vi "IMAQdx Low-Level Grab Async with AVI Recording LV2012 NIVerified.vi"() -> ()   [LabVIEW 2012]
doc: "Demonstrates how to save acquired images to a AVI.\n\nIn this example a IMAQdx Acquisition (e.g. USB Webcams) is used to generate images that can be saved to a AVI file. But in general a AVI file can be generated off every series of IMAQ Images. Other IMAQ Image sources could be other IMAQ drivers (IMAQ, IMAQ I/O) or loading a series of images from disk."
uses:
  <vilib>/userdefined/High Color/IMAQdx.ctl
  <vilib>/vision/driver/IMAQdx.llb/IMAQdx Acquisition Mode.ctl
  <vilib>/vision/driver/IMAQdx.llb/IMAQdx Buffer Number Mode.ctl
  <vilib>/vision/driver/NI_Vision_Acquisition_Software.lvlib
  <resource>/objmgr/imaqdx.rc
panel:
  in  "stop":bool
  in  "Record":bool
  in  "Camera Name":T1
  out "Image":T2(plugin-control)
  out "Buffer Number":u32
  out "Event Overrun":bool
  in  "AVI File Path":path
  # "Overview: Demonstrates how to save acquired images to a AVI video\nRequirements: LabVIEW 2012 Base Development System  (or compatible)\n                             Vision Development Module 2012 (or compatible)\n                             NI-IMAQdx 4.0 (or compatible)\nInstructions: \n1. Select the path to the AVI file\n2. Select the camera name\n3. Run the VI\n4. Activate the Record button to start writing image frames to the AVI\n5. Release the button to stop recording"
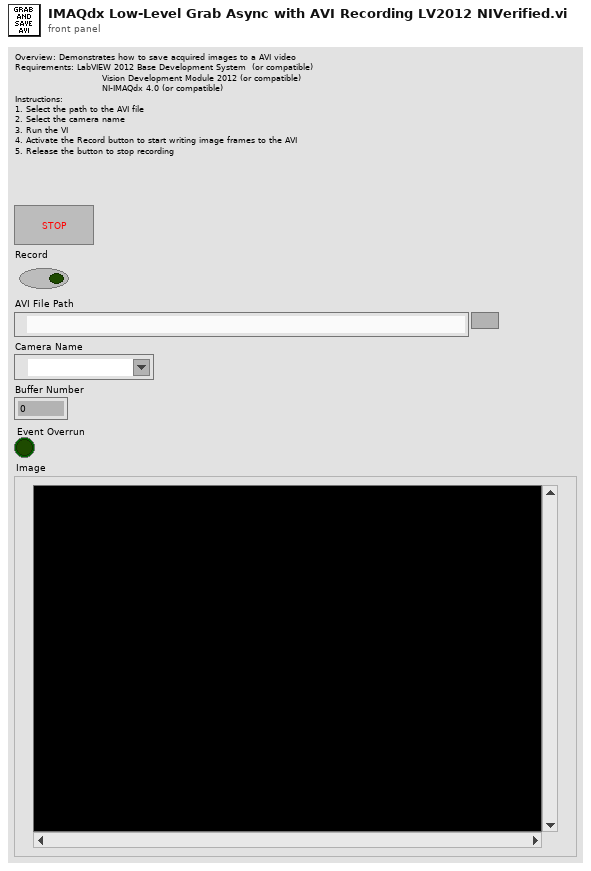
[diagram p1: front panel]
types:
  T1 = typedef "IMAQdx.ctl" = refnum<k21>
  T2 = typedef "IMAQ Image.ctl" = refnum<image>
  T3 = typedef "NI_Vision_Acquisition_Software.lvlib/IMAQdx Acquisition Mode.ctl" = enum32{"One Shot", "Continuous"}
  T4 = typedef "IMAQ AVI2 Refnum.ctl" = refnum<k20>
  T5 = typedef "NI_Vision_Acquisition_Software.lvlib/IMAQdx Buffer Number Mode.ctl" = enum32{"Next", "Last", "Buffer Number"}
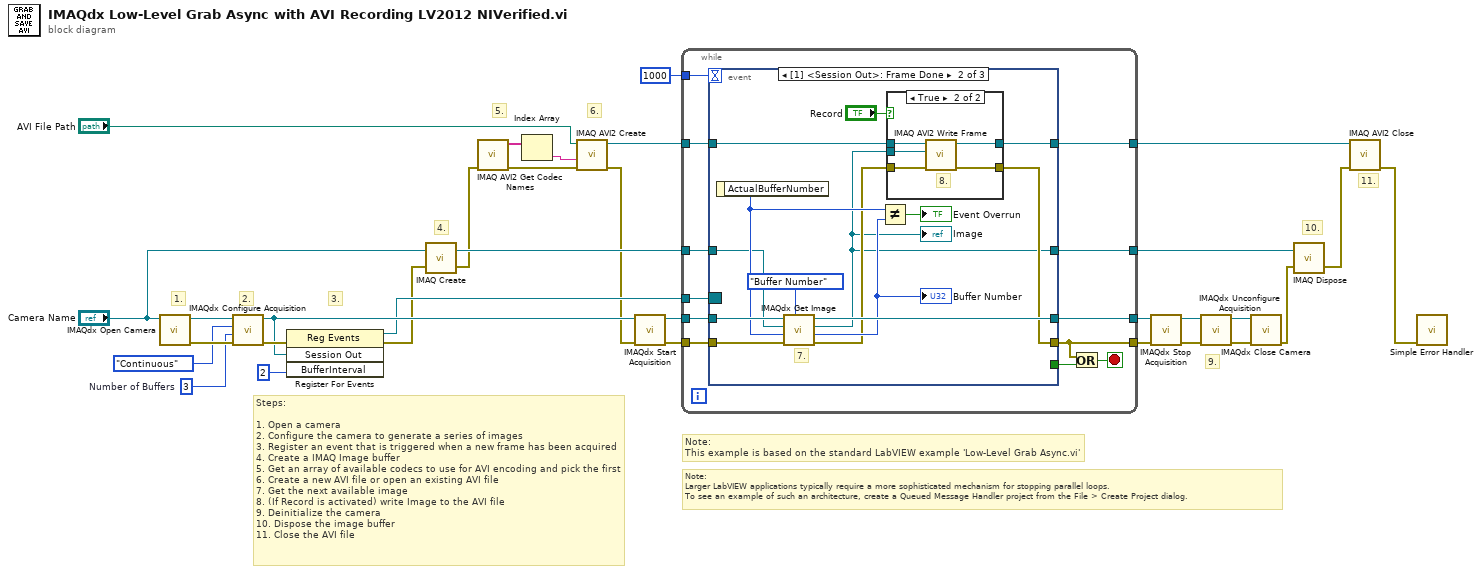
[diagram p0: block diagram]
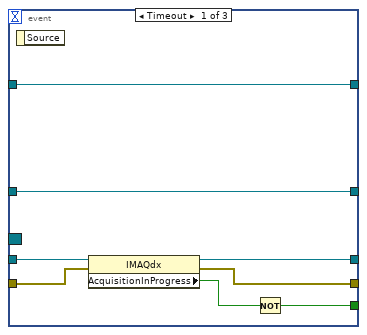
[diagram p2: hidden frame]
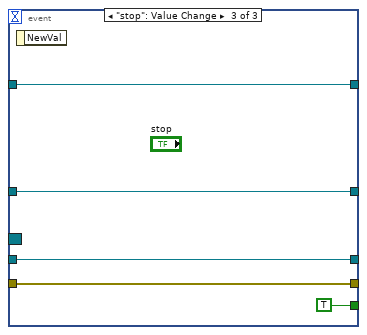
[diagram p4: hidden frame]
diagram:
  w26 = u32 3  # Number of Buffers
  # "Note:\nLarger LabVIEW applications typically require a more sophisticated mechanism for stopping parallel loops.\nTo see an example of such an architecture, create a Queued Message Handler project from the File > Create Project dialog."
  # "10."
  # "11."
  # "9."
  # "6."
  # "5."
  # "4."
  # "3."
  # "2."
  # "1."
  # "Note:\nThis example is based on the standard LabVIEW example 'Low-Level Grab Async.vi'"
  # "Steps:\n\n1. Open a camera\n2. Configure the camera to generate a series of images \n3. Register an event that is triggered when a new frame has been acquired\n4. Create a IMAQ Image buffer\n5. Get an array of available codecs to use for AVI encoding and pick the first\n6. Create a new AVI file or open an existing AVI file\n7. Get the next available image\n8. (If Record is activated) write Image to the AVI file\n9. Deinitialize the camera\n10. Dispose the image buffer\n11. Close the AVI file"
  n1 = call <vilib>:"IMAQdx Open Camera.vi"("Session In"="Camera Name") -> ("error out"=w28:errorcluster, "Session Out"=w30:T1)  [unwired: 2 in, 7 out]
  n2 = call <vilib>:"IMAQdx Configure Acquisition.vi"("error in"=w28, "Number of Buffers"=w26, "Continuous?"=IMAQdx_Acquisition_Mode."Continuous", "Session In"=w30) -> ("error out"=w19:errorcluster, "Session Out"=w18:T1)  [unwired: 6 out]
  n3 = register-events(error in=w19, w18, u32 2 ("BufferInterval")) -> (reference out=w16:refnum<event-registration>, error out=w14:errorcluster)  [unwired: 1 in]
  n4 = call "IMAQ Create"("Image Name"="Camera Name", "error in (no error)"=w14) -> ("New Image"=w32:T2, "error out"=w13:errorcluster)  [unwired: 2 in, 1 out]
  n5 = call "IMAQ AVI2 Get Codec Names"("error in (no error)"=w13) -> ("error out"=w9:errorcluster, "Codec Names"=w12:string[])  [unwired: 9 in]
  n6 = Index Array(array=w12) -> (element=w10:string)  [unwired: 1 in]
  n7 = call "IMAQ AVI2 Create"("error in (no error)"=w9, "Codec"=w10, "AVI Path"="AVI File Path") -> ("error out"=w7:errorcluster, "AVI Refnum"=w6:T4)  [unwired: 7 in]
  n8 = call <vilib>:"IMAQdx Start Acquisition.vi"("error in"=w7, "Session In"=w18) -> ("error out"=w8:errorcluster, "Session Out"=w29:T1)  [unwired: 8 out]
  n9 = while {
    tunnel: [w40] -> w24
    tunnel: w8 -> [w42]
    tunnel: w29 -> [w43]
    tunnel: [w37] -> w25
    tunnel: w32 -> [w41]
    tunnel: w16 -> [w39]
    tunnel: 1000 -> [w38]
    tunnel: w6 -> [w35]
    tunnel: [w34] -> w5
    tunnel: [w33] -> w3
    stop <- w44 stop-if-true
    n10 = event shown="[1] <Session Out>: Frame Done" {
      selector: w39 -> [_ _ _]
      dyn-events: _ -> [_ _ _]
      timeout: w38 -> [_ _ _]
      tunnel: w43 -> [w52 w66 w77]
      tunnel: w42 -> [w48 w65 w78]
      tunnel: w41 -> [w50 w54 w74]
      tunnel: [w49 w64 w77] -> w40
      tunnel: [w47 w56 w78] -> w37
      tunnel: [w45 _ TRUE] -> w36
      tunnel: w35 -> [w51 w59 w75]
      tunnel: [w51 w58 w75] -> w34
      tunnel: [w50 w53 w74] -> w33
      event Timeout {
        n11 = event-data() -> ()  [unwired: 2 out]
        n12 = property class="IMAQdx"(reference=w52, error in=w48) -> (reference out=w49:T1, error out=w47:errorcluster, "AcquisitionInProgress"=w46:bool)
        n13 = Not(x=w46) -> (.not. x?=w45:bool)
      }
      event event #0x0 {
        # "7."
        n14 = event-data() -> ("ActualBufferNumber"=w62:u32)  [unwired: 1 out]
        n15 = call <vilib>:"IMAQdx Get Image.vi"("Buffer Number Mode (Next)"=IMAQdx_Buffer_Number_Mode."Buffer Number" ("Buffer Number Mode"), "error in"=w65, "Buffer Number In"=w62, "Image In"=w54, "Session In"=w66) -> ("error out"=w57:errorcluster, "Buffer Number Out"=w61:u32, "Image Out"=w53:T2, "Session Out"=w64:T1)  [unwired: 3 out]
        "Image" <- w53
        "Buffer Number" <- w61
        n16 = Not Equal?(x=w62, y=w61) -> (x != y?=→"Event Overrun":bool)
        n17 = case shown="True" "Record" {
          tunnel: w59 -> [w67 w73]
          tunnel: [w67 w72] -> w58
          tunnel: w53 -> [_ w71]
          tunnel: w57 -> [w68 w70]
          tunnel: [w68 w69] -> w56
          frame False {
          }
          frame True {
            # "8."
            n18 = call "IMAQ AVI2 Write Frame"("error in (no error)"=w70, "Image"=w71, "AVI Refnum"=w73) -> ("error out"=w69:errorcluster, "AVI Refnum (duplicate)"=w72:T4)  [unwired: 6 in, 1 out]
          }
        }
      }
      event "stop": Value Change {
        n19 = event-data() -> ()  [unwired: 2 out]
      }
    }
    n20 = Or(x=w37, y=w36) -> (x .or. y?=w44:bool)
  }
  n21 = call <vilib>:"IMAQdx Stop Acquisition.vi"("error in"=w25, "Session In"=w24) -> ("error out"=w20:errorcluster, "Session Out"=w21:T1)  [unwired: 8 out]
  n22 = call <vilib>:"IMAQdx Unconfigure Acquisition.vi"("error in"=w20, "Session In"=w21) -> ("error out"=w23:errorcluster, "Session Out"=w22:T1)  [unwired: 8 out]
  n23 = call <vilib>:"IMAQdx Close Camera.vi"("error in"=w23, "Session In"=w22) -> ("error out"=w2:errorcluster)  [unwired: 9 out]
  n24 = call "IMAQ Dispose"("Image"=w3, "error in (no error)"=w2) -> ("error out"=w1:errorcluster)  [unwired: 4 in]
  n25 = call "IMAQ AVI2 Close"("error in (no error)"=w1, "AVI Refnum"=w5) -> ("error out"=w4:errorcluster)  [unwired: 9 in]
  n26 = call <vilib>:"Simple Error Handler.vi"("error in (no error)"=w4) -> ()  [unwired: 4 in, 5 out]
